vi "set_config_cluster.vi"(8 "error in (no error)":errorcluster, 10 "config cluster variant":variant, 11 "GenericPlugin in":refnum<class "StageMH110930Scientifica.lvclass">) -> (0 "error out":errorcluster, 3 "GenericPlugin out":refnum<class "StageMH110930Scientifica.lvclass">)   [LabVIEW 2010, in "StageMH110930Scientifica.lvclass"]
uses:
  StageMH110930Scientifica.lvclass
  StageMH110930Scientifica.lvclass/StageMH110930Scientifica.ctl
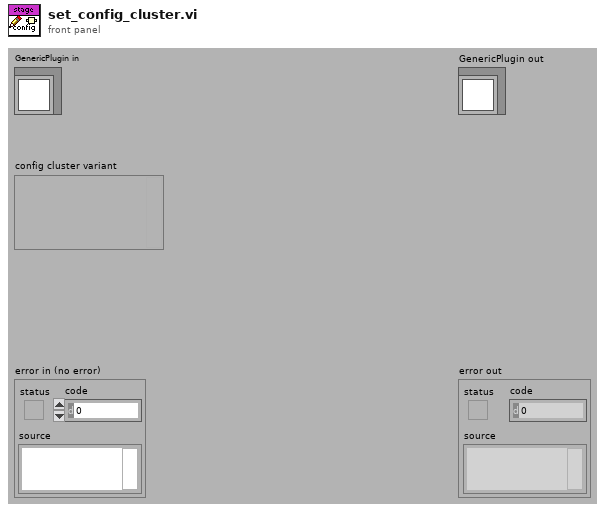
[diagram p1: front panel]
types:
  T1 = typedef "StageMH110930Scientifica.lvclass/config_data_cluster.ctl" = cluster{"serial port name":refnum<visa-resource-name>}
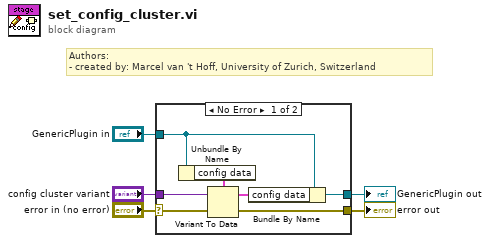
[diagram p0: block diagram]
diagram:
  # "Authors: \n- created by: Marcel van 't Hoff, University of Zurich, Switzerland"
  n1 = case shown="No Error" "error in (no error)" {
    selector: "error in (no error)" -> [w10 w13]
    tunnel: "GenericPlugin in" -> [w6 w14]
    tunnel: [w8 w13] -> w2
    tunnel: [w7 w14] -> w1
    tunnel: "config cluster variant" -> [w9 _]
    frame No Error {
      n2 = Unbundle By Name(w6) -> ("config data"=w12:T1)
      n3 = Variant To Data(error in=w10, Variant=w9, type=w12) -> (error out=w8:errorcluster, data=w11:T1)
      n4 = Bundle By Name(cluster=w6, "config data"=w11) -> (w7:refnum<class "StageMH110930Scientifica.lvclass">)
    }
    frame Error {
    }
  }
  "error out" <- w2
  "GenericPlugin out" <- w1
